vi "Page_Source_Can_Add_To_Bottom.vi"(8 "error in (no error)":errorcluster, 11 "AB_Source_Container in":refnum<class "AB_Source_Container.lvclass">) -> (0 "error out":errorcluster, 1 "message":string, 2 "canAddToBottom":bool, 3 "AB_Source_Container out":refnum<class "AB_Source_Container.lvclass">)   [LabVIEW 2020, in "AB_Source_Container.lvclass"]
uses:
  <vilib>/AppBuilder/AB_Classes/Source/Container/AB_Source_Container.lvclass
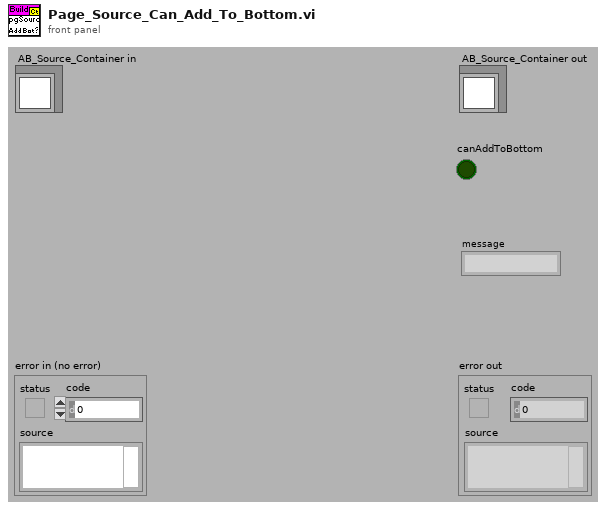
[diagram p1: front panel]
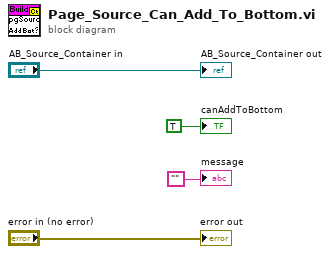
[diagram p0: block diagram]
diagram:
  "error out" <- "error in (no error)"
  "canAddToBottom" <- TRUE ("canAdd")
  "AB_Source_Container out" <- "AB_Source_Container in"
  "message" <- ""
